vi "EnqueueElement.vi"(6 "AtOpposite":bool, 8 "error in (no error)":errorcluster, 9 "Data":variant[](array[variant]), 10 "Actions":string[](array[string]), 11 "QueueIN":refnum<queue>) -> (0 "error out":errorcluster, 3 "QueueOUT":refnum<queue>)   [LabVIEW 2018]
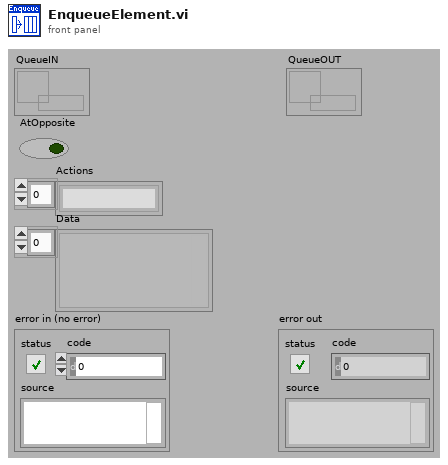
[diagram p1: front panel]
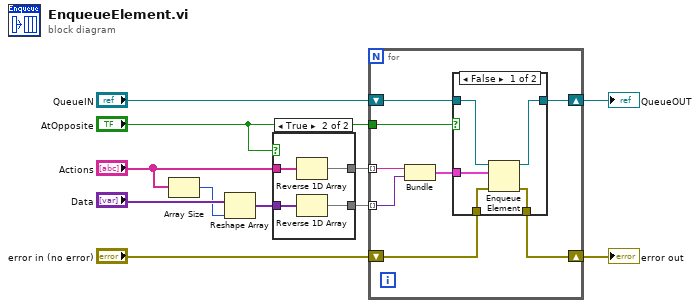
[diagram p0: block diagram]
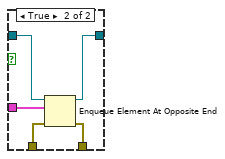
[diagram p3: hidden frame]
diagram:
  n1 = Array Size(array="Actions") -> (size(s)=w8:i32)
  n2 = Reshape Array("Data", w8) -> (w9:variant[])
  n3 = case shown="True" "AtOpposite" {
    tunnel: "Actions" -> [w13 w17]
    tunnel: w9 -> [w12 w16]
    tunnel: [w13 w15] -> w5
    tunnel: [w12 w14] -> w4
    frame False {
    }
    frame True {
      n4 = Reverse 1D Array(array=w17) -> (reversed array=w15:string[])
      n5 = Reverse 1D Array(array=w16) -> (reversed array=w14:variant[])
    }
  }
  n6 = for {
    tunnel: "AtOpposite" -> [w25]
    tunnel: w5 -> [w22] mode=indexing
    tunnel: w4 -> [w21] mode=indexing
    shift-right: [w19] -> w1
    shift-left: "error in (no error)" -> [w23]
    shift-right: [w18] -> w3
    shift-left: "QueueIN" -> [w24]
    n7 = Bundle("字符串"=w22, "变体"=w21) -> (w20:cluster{"字符串":string, "变体":variant})  [unwired: 1 out]
    n8 = case shown="False" w25 {
      tunnel: w24 -> [w29 w35]
      tunnel: w23 -> [w28 w34]
      tunnel: w20 -> [w30 w33]
      tunnel: [w27 w31] -> w19
      tunnel: [w26 w32] -> w18
      frame False {
        n9 = Enqueue Element(queue=w29, element=w30, error in (no error)=w28) -> (queue out=w26:refnum<queue>, error out=w27:errorcluster)  [unwired: 2 out]
      }
      frame True {
        n10 = Enqueue Element At Opposite End(queue=w35, element=w33, error in (no error)=w34) -> (queue out=w32:refnum<queue>, error out=w31:errorcluster)  [unwired: 2 out]
      }
    }
  }
  "QueueOUT" <- w3
  "error out" <- w1
